vi "_create_array_command.vi"(8 "error in":errorcluster, 9 "precision (1)":i16=1, 10 "array":dbl[](array[numeric]), 11 "Command in":string) -> (0 "error out":errorcluster, 3 "Command out":string)   [LabVIEW 2016, in "Chemyx_Syringe_Pump_driver.lvlib"]
doc: "Appends a string created from an array of double floats values to Command in. Each value is converted to a floating point representation using the precision input for the number of digits. The Resulting string isoutput as Command out.\n\nPrivate VI."
uses:
  Chemyx_Syringe_Pump_driver.lvlib
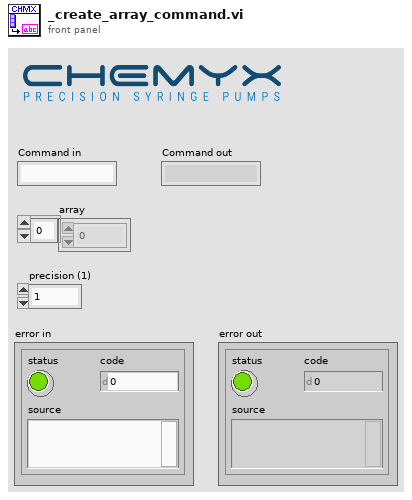
[diagram p1: front panel]
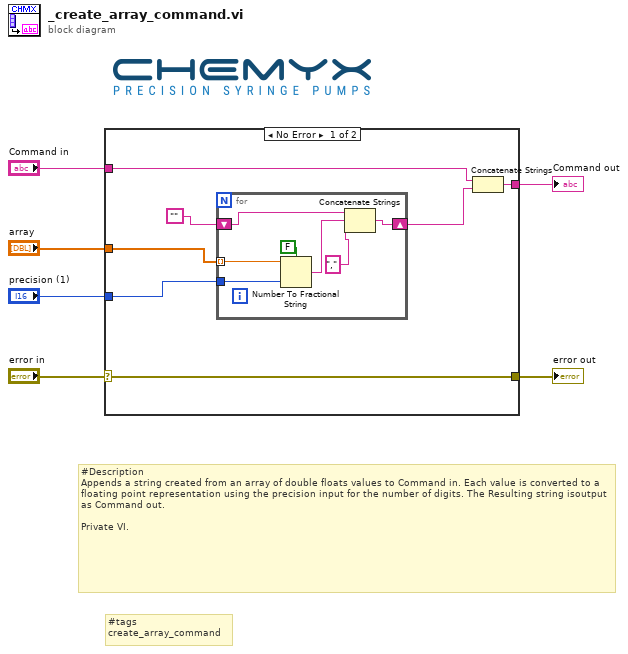
[diagram p0: block diagram]
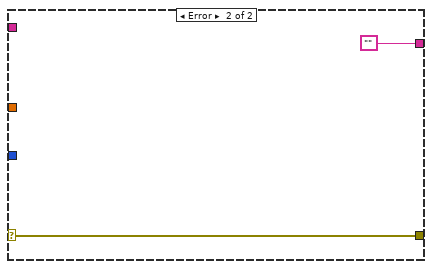
[diagram p2: hidden frame]
diagram:
  # "#tags\ncreate_array_command"
  # "#Description\nAppends a string created from an array of double floats values to Command in. Each value is converted to a floating point representation using the precision input for the number of digits. The Resulting string isoutput as Command out.\n\nPrivate VI."
  n1 = case shown="No Error" "error in" {
    selector: "error in" -> [w7 w22]
    tunnel: "precision (1)" -> [w13 _]
    tunnel: "array" -> [w10 _]
    tunnel: [w9 ""] -> w4
    tunnel: "Command in" -> [w8 _]
    tunnel: [w7 w22] -> w1
    frame No Error {
      n2 = for {
        tunnel: w10 -> [w20] mode=indexing
        shift-right: [w18] -> w12
        shift-left: "" -> [w17]
        tunnel: w13 -> [w14]
        n3 = Number To Fractional String(use system decimal point (T)=FALSE, number=w20, precision (6)=w14) -> (F-format string=w16:string)  [unwired: 1 in]
        n4 = Concatenate Strings(w17, w16, ",") -> (w18:string)
      }
      n5 = Concatenate Strings(w8, w12) -> (w9:string)
    }
    frame Error {
    }
  }
  "Command out" <- w4
  "error out" <- w1
